vi "Set Numeric Without Type Preservation.vi"(10 "Numeric":i32, 11 "Parent in":refnum<class "Parent.lvclass">) -> (3 "Parent out":refnum<class "Parent.lvclass">)   [LabVIEW 2023, in "Parent.lvclass"]
doc: "In this VI, the Parent object does not propagate from the input to the output terminal."
uses:
  Parent.lvclass
  Child/Child.lvclass
  c:/dev/_r/4/eng/lv-core/lvpostprocessingd/lv_mc_x86_64/dist_i386/examples/Object-Oriented Programming/Preserve Run-Time Class/Parent/Parent.lvclass
  Parent.lvclass/Parent.ctl
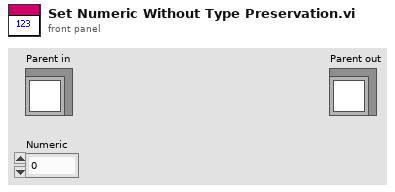
[diagram p1: front panel]
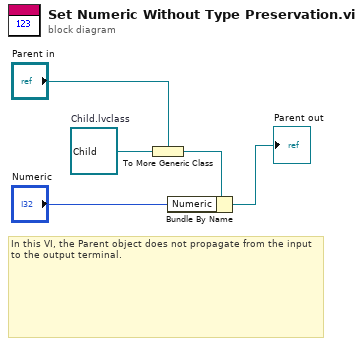
[diagram p0: block diagram]
diagram:
  w3 = refnum<class "Child.lvclass"> refnum  # Child.lvclass
  # "In this VI, the Parent object does not propagate from the input to the output terminal."
  n1 = To More Generic Class(target class="Parent in", reference=w3) -> (generic class reference=w1:refnum<class "Parent.lvclass">)
  n2 = Bundle By Name(cluster=w1, "Numeric"="Numeric") -> (→"Parent out":refnum<class "Parent.lvclass">)
